vi "test-importValue.vi"() -> ()   [LabVIEW 2019, in "lv-apt-json-file-test.lvlib"]
uses:
  lv-apt-json-file-test.lvlib
  src/Typedef/Def-AttrMap.ctl
panel:
  in  "Tree 2":string(tree)
  in  "Tree":string(tree)
  out "OrignKey":string
  out "Variant":variant
  out "AttrMap out":T1
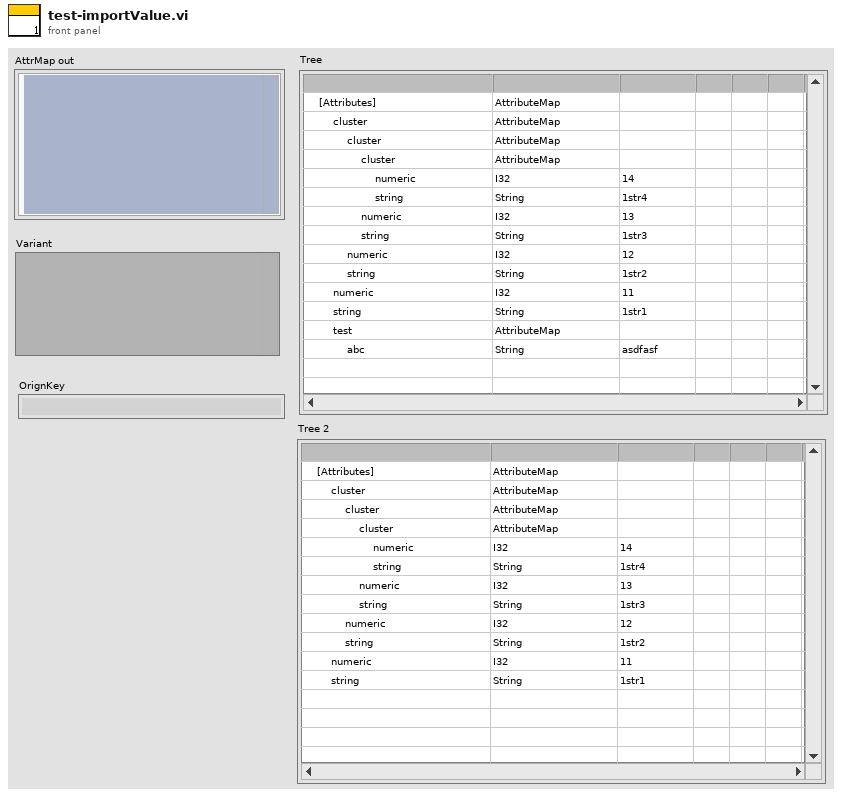
[diagram p1: front panel]
types:
  T1 = typedef "Def-AttrMap.ctl" = cluster{"Map":variant}
  T2 = cluster{"nUmeric":i32, "string":string, "Cluster":cluster{"numeric":i32, "string":string, "cluster":cluster{"numeric":i32, "string":string, "cluster":cluster{"numeric":i32, "string":string}}}}
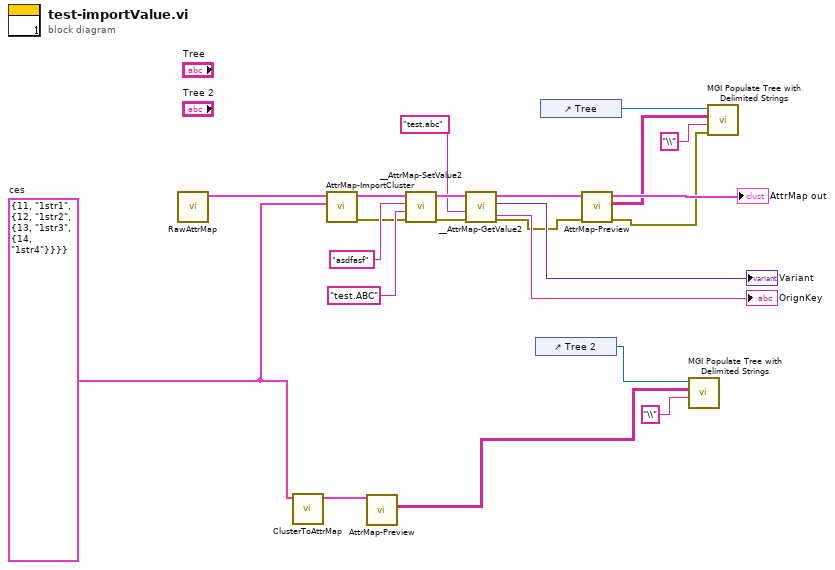
[diagram p0: block diagram]
diagram:
  w4 = T2 {"nUmeric"=11, "string"="1str1", "Cluster"={"numeric"=12, "string"="1str2", "cluster"={"numeric"=13, "string"="1str3", "cluster"={"numeric"=14, "string"="1str4"}}}}  # ces
  n1 = call "RawAttrMap.vi"() -> ("AttrMap"=w12:T1)  [unwired: 11 in]
  n2 = call "ClusterToAttrMap.vi"("data"=w4) -> ("AttrMap"=w5:T1)  [unwired: 9 in, 1 out]
  n3 = call "AttrMap-ImportCluster.vi"("Cluster"=w4, "AttrMap in"=w12) -> ("error out"=w10:errorcluster, "AttrMap out"=w11:T1)  [unwired: 8 in]
  n4 = call "AttrMap-Preview.vi"("AttrMap in"=w5) -> ("table"=w2:string[][])  [unwired: 8 in, 2 out]
  n5 = call "__AttrMap-SetValue2.vi"("error in (no error)"=w10, "Key"="test.ABC", "Value"="asdfasf", "AttrMap in"=w11) -> ("error out"=w13:errorcluster, "AttrMap out"=w22:T1)  [unwired: 6 in]
  n6 = call "__AttrMap-GetValue2.vi"("error in (no error)"=w13, "Key"="test.abc", "AttrMap in"=w22) -> ("error out"=w14:errorcluster, "VAttributes"=→"Variant":variant, "AttrMap out"=w19:T1, "OrignKey"=→"OrignKey":string)  [unwired: 4 in, 1 out]
  n7 = control-ref of="Tree 2"() -> (w1:refnum<vi>)
  n8 = control-ref of="Tree"() -> (w8:refnum<vi>)
  n9 = call "AttrMap-Preview.vi"("error in (no error)"=w14, "AttrMap in"=w19) -> ("error out"=w6:errorcluster, "table"=w9:string[][], "AttrMap out"=→"AttrMap out":T1)  [unwired: 7 in]
  n10 = call <userlib>:"MGI Populate Tree with Delimited Strings.vi"("Delimiter"="\\", "Items (Delimited)"=w2, "Tree Control"=w1) -> ()  [unwired: 6 in, 3 out]
  n11 = call <userlib>:"MGI Populate Tree with Delimited Strings.vi"("error in (no error)"=w6, "Delimiter"="\\", "Items (Delimited)"=w9, "Tree Control"=w8) -> ()  [unwired: 5 in, 3 out]
